vi "MessageReceiver.vi"() -> ()   [LabVIEW 2018]
uses:
  <vilib>/myRIO/Instrument Drivers/Onboard IO/AI/typedefs/AI Reference.ctl
  <vilib>/myRIO/Common/Instrument Driver Framework/Utilities/typedefs/myRIO Generic Hardware Reference.ctl
  <vilib>/myRIO/Common/Instrument Driver Framework/Utilities/typedefs/Hardware Version Enum.ctl
  <vilib>/myRIO/Common/Instrument Driver Framework/Utilities/typedefs/myRIO v1.0 Reference.ctl
  <vilib>/myRIO/Common/Instrument Driver Framework/Utilities/typedefs/Generic FPGA Reference.ctl
  <vilib>/myRIO/Common/Instrument Driver Framework/myRIO v1.0/AI/typedefs/AI Channels List.ctl
  <vilib>/myRIO/Common/Instrument Driver Framework/myRIO v1.0/AI/typedefs/AI Channels Enum.ctl
  <vilib>/myRIO/Common/Instrument Driver Framework/Utilities/typedefs/Analog Scaling Constants List.ctl
  <vilib>/myRIO/Common/Instrument Driver Framework/Utilities/typedefs/Analog Scaling Constants.ctl
  <vilib>/userdefined/High Color/nirio_resource_hc.ctl
  <vilib>/myRIO/Common/Instrument Driver Framework/ELVIS III v1.0/AI/vis/ELVIS III v1.1 Open AI.vi
  <vilib>/myRIO/Common/Instrument Driver Framework/Utilities/vis/Validate Channels.vi
  <vilib>/myRIO/Common/Instrument Driver Framework/ELVIS III v1.0/AI/vis/ELVIS III v1.0 Reserve AI.vi
  <vilib>/myRIO/Common/Instrument Driver Framework/ELVIS III v1.0/AI/vis/ELVIS III v1.0 Close AI.vi
  <vilib>/myRIO/Common/Instrument Driver Framework/ELVIS III v1.0/Resource Manager/vis/ELVIS III v1.0 Reserve Channel List.vi
  <vilib>/myRIO/Common/Instrument Driver Framework/ELVIS III v1.0/AI/vis/ELVIS III v1.0 Build MUX Configuration AI.vi
  <vilib>/myRIO/Common/Instrument Driver Framework/ELVIS III v1.0/AI/vis/ELVIS III v1.0 Unreserve AI.vi
  <vilib>/myRIO/Common/Instrument Driver Framework/ELVIS III v1.0/Resource Manager/vis/ELVIS III v1.0 Reserve Channel.vi
  <vilib>/myRIO/Common/Instrument Driver Framework/ELVIS III v1.0/Resource Manager/vis/ELVIS III v1.0 Unreserve Channel.vi
  <vilib>/myRIO/Common/Instrument Driver Framework/ELVIS III v1.0/Resource Manager/vis/ELVIS III v1.0 Unreserve Channel List.vi
  <vilib>/myRIO/Common/Instrument Driver Framework/ELVIS III v1.0/Resource Manager/vis/ELVIS III v1.0 Build Mutex Name.vi
  <vilib>/Utility/VariantDataType/GetNumericInfo.vi
  <vilib>/Utility/error.llb/Error Cluster From Error Code.vi
  <vilib>/myRIO/Common/Instrument Driver Framework/ELVIS III v1.0/ELVIS III v1.1 Open.vi
  <vilib>/myRIO/Common/Instrument Driver Framework/ELVIS III v1.0/Resource Manager/vis/ELVIS III v1.0 Coerce AI Scaling.vi
  <vilib>/myRIO/Common/Instrument Driver Framework/Utilities/vis/IO Manager.vi
  <vilib>/myRIO/Common/Instrument Driver Framework/Utilities/vis/Configuration Manager.vi
  <vilib>/myRIO/Common/Instrument Driver Framework/ELVIS III v1.0/Resource Manager/vis/ELVIS III v1.0 Configure AI Mode.vi
  <vilib>/myRIO/Common/Instrument Driver Framework/myRIO v1.0/myRIO v1.0 Close.vi
  <vilib>/myRIO/Common/Instrument Driver Framework/ELVIS III v1.0/AI/vis/ELVIS III v1.0 Read AI.vi
  <vilib>/myRIO/Instrument Drivers/Onboard IO/AI/vis/myRIO AI Open.xnode
  <vilib>/myRIO/Instrument Drivers/Onboard IO/AI/AI.lvlib
panel:
  in  "Stop Button":bool
  out "Current State":string
  out "Total String Read":string
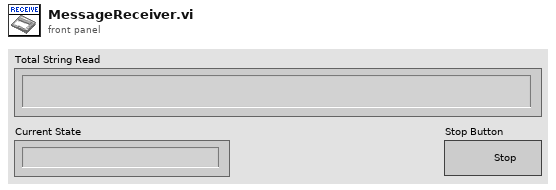
[diagram p1: front panel]
types:
  T1 = enum16{"Waiting to Acquire", "Processing", "Acquire"}
  T2 = typedef "AI.lvlib/AI Reference.ctl" = cluster{"myRIO Reference":T3, "AI Channels List":T7, "AI Scaling Constants List":T9}
  T3 = typedef "myRIO Generic Hardware Reference.ctl" = cluster{"myRIO Model":T4, "myRIO Hardware Reference":T5}
  T4 = typedef "Hardware Version Enum.ctl" = enum16{"Unknown", "myRIO-1900", "myRIO-1950", "roboRIO", "NI ELVIS RIO CM", "ELVIS III"}
  T5 = typedef "myRIO v1.0 Reference.ctl" = cluster{"Generic FPGA Reference":T6, "Allow multiple opens":bool}
  T6 = typedef "Generic FPGA Reference.ctl" = refnum<k20>
  T7 = typedef "AI Channels List.ctl" = T8[]
  T8 = typedef "AI Channels Enum.ctl" = enum16{"Not Connected", "AudioIn/Left", "AudioIn/Right", "C/AI0", "C/AI1", "A/AI0", "A/AI1", "A/AI2", "A/AI3", "A/AI4", "A/AI5", "A/AI6", "A/AI7", "B/AI0", "B/AI1", "B/AI2", "B/AI3", "B/AI4", "B/AI5", "B/AI6", "B/AI7", "AI/AI0", "AI/AI1", "AI/AI2", "AI/AI3", "A/AI0 (DIFF)", "A/AI1 (DIFF)", "A/AI2 (DIFF)", "A/AI3 (DIFF)", "B/AI0 (DIFF)", "B/AI1 (DIFF)", "B/AI2 (DIFF)", "B/AI3 (DIFF)"}
  T9 = typedef "Analog Scaling Constants List.ctl" = T10[]
  T10 = typedef "Analog Scaling Constants.ctl" = cluster{"LSB Weight (Volts)":dbl, "Offset (Volts)":dbl, "Signed?":bool}
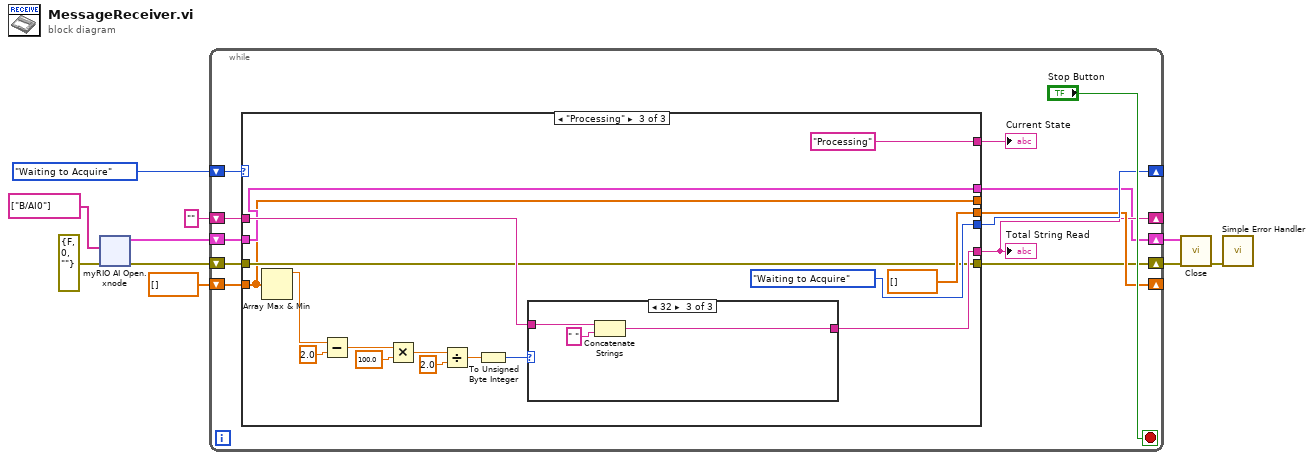
[diagram p0: block diagram]
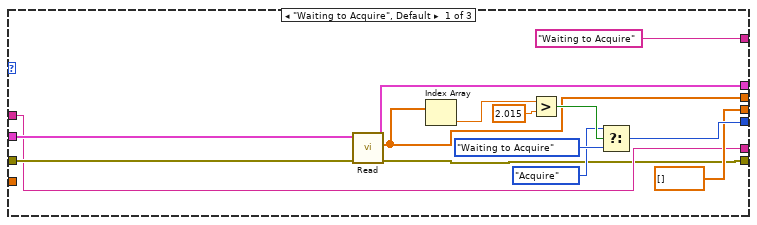
[diagram p2: hidden frame]
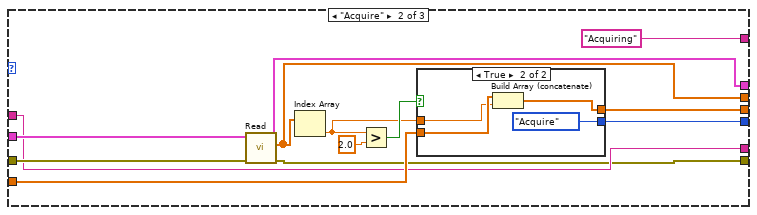
[diagram p3: hidden frame]
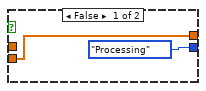
[diagram p4: hidden frame]
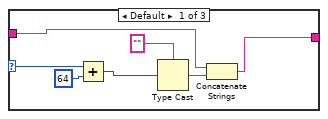
[diagram p5: hidden frame]
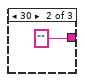
[diagram p6: hidden frame]
diagram:
  n1 = xnode "myRIO AI Open.xnode"("error in (no error)"=errorcluster {"status"=FALSE, "code"=0, "source"=""}, "Channel Names"=tag[] ["B/AI0"]) -> ("error out"=w10:errorcluster, "AI Ref Out"=w9:T2)  [unwired: 3 in]
  n2 = while {
    shift-right: [w19] -> _
    shift-left: T1."Waiting to Acquire" -> [w16]
    shift-right: [w18] -> _
    shift-left: dbl[] [] -> [w17]
    shift-right: [w13] -> _
    shift-left: "" -> [w14]
    shift-right: [w12] -> w8
    shift-left: w9 -> [w21]
    shift-right: [w11] -> w7
    shift-left: w10 -> [w20]
    stop <- "Stop Button" stop-if-true
    n3 = case shown="\"Processing\"" w16 {
      tunnel: w21 -> [w36 w49 w58]
      tunnel: w20 -> [w35 w48 w57]
      tunnel: [w32 w43 T1."Waiting to Acquire"] -> w19
      tunnel: [dbl[] [] w44 dbl[] []] -> w18
      tunnel: w17 -> [_ w47 w56]
      tunnel: ["Waiting to Acquire" "Acquiring" "Processing"] -> w15
      tunnel: w14 -> [w26 w40 w61]
      tunnel: [w26 w40 w60] -> w13
      tunnel: [w25 w39 w58] -> w12
      tunnel: [w24 w38 w57] -> w11
      tunnel: [w23 w37 w56] -> _
      frame "Waiting to Acquire", Default {
        n4 = call <vilib>:"Read.vi"("error in (no error)"=w35, "AI Ref In"=w36) -> ("error out"=w24:errorcluster, "Values"=w23:dbl[], "AI Ref Out"=w25:T2)  [unwired: 7 in]
        n5 = Index Array(array=w23) -> (element=w27:dbl)  [unwired: 1 in]
        n6 = Greater?(x=w27, y=2.015) -> (0:w33:bool)
        n7 = Select(t=T1."Acquire", s=w33, f=T1."Waiting to Acquire") -> (s? t:f=w32:T1)
      }
      frame "Acquire" {
        n8 = call <vilib>:"Read.vi"("error in (no error)"=w48, "AI Ref In"=w49) -> ("error out"=w38:errorcluster, "Values"=w37:dbl[], "AI Ref Out"=w39:T2)  [unwired: 7 in]
        n9 = Index Array(array=w37) -> (element=w41:dbl)  [unwired: 1 in]
        n10 = Greater?(x=w41, y=2.0) -> (0:w45:bool)
        n11 = case shown="True" w45 {
          tunnel: w47 -> [w51 w55]
          tunnel: [w51 w54] -> w44
          tunnel: [T1."Processing" T1."Acquire"] -> w43
          tunnel: w41 -> [_ w52]
          frame False {
          }
          frame True {
            n12 = Build Array (concatenate)(w55, w52) -> (w54:dbl[])
          }
        }
      }
      frame "Processing" {
        n13 = Array Max & Min(array=w56) -> (max value=w69:dbl)  [unwired: 3 out]
        n14 = Subtract(x=w69, y=2.0) -> (x-y=w67:dbl)
        n15 = Multiply(x=w67, y=100.0) -> (x*y=w65:dbl)
        n16 = Divide(x=w65, y=2.0) -> (x/y=w63:dbl)
        n17 = To Unsigned Byte Integer(number=w63) -> (unsigned 8bit integer=w59:u8)
        n18 = case shown="32" w59 {
          selector: w59 -> [w72 _ _]
          tunnel: w61 -> [w73 _ w82]
          tunnel: [w74 "" w80] -> w60
          frame Default {
            n19 = Add(x=w72, y=u8 64) -> (x+y=w77:u8)
            n20 = Type Cast(type="", x=w77) -> (*(type *) &x=w75:string)
            n21 = Concatenate Strings(w73, w75) -> (w74:string)
          }
          frame 30 {
          }
          frame 32 {
            n22 = Concatenate Strings(w82, " ") -> (w80:string)
          }
        }
      }
    }
    "Current State" <- w15
    "Total String Read" <- w13
  }
  n23 = call <vilib>:"Close.vi"("error in (no error)"=w7, "AI Ref In"=w8) -> ("error out"=w2:errorcluster)  [unwired: 9 in]
  n24 = call <vilib>:"Simple Error Handler.vi"("error in (no error)"=w2) -> ()  [unwired: 4 in, 5 out]
